vi "PNGout.vi"(2 "PNG file path":path=path "/Users/leogallacio/Downloads/N8.png", 7 "Paths error":errorcluster) -> (13 "PNGRead error":errorcluster, 14 "PNG picture":picture, 15 "Width":i16, 16 "Height":i16)   [LabVIEW 2023]
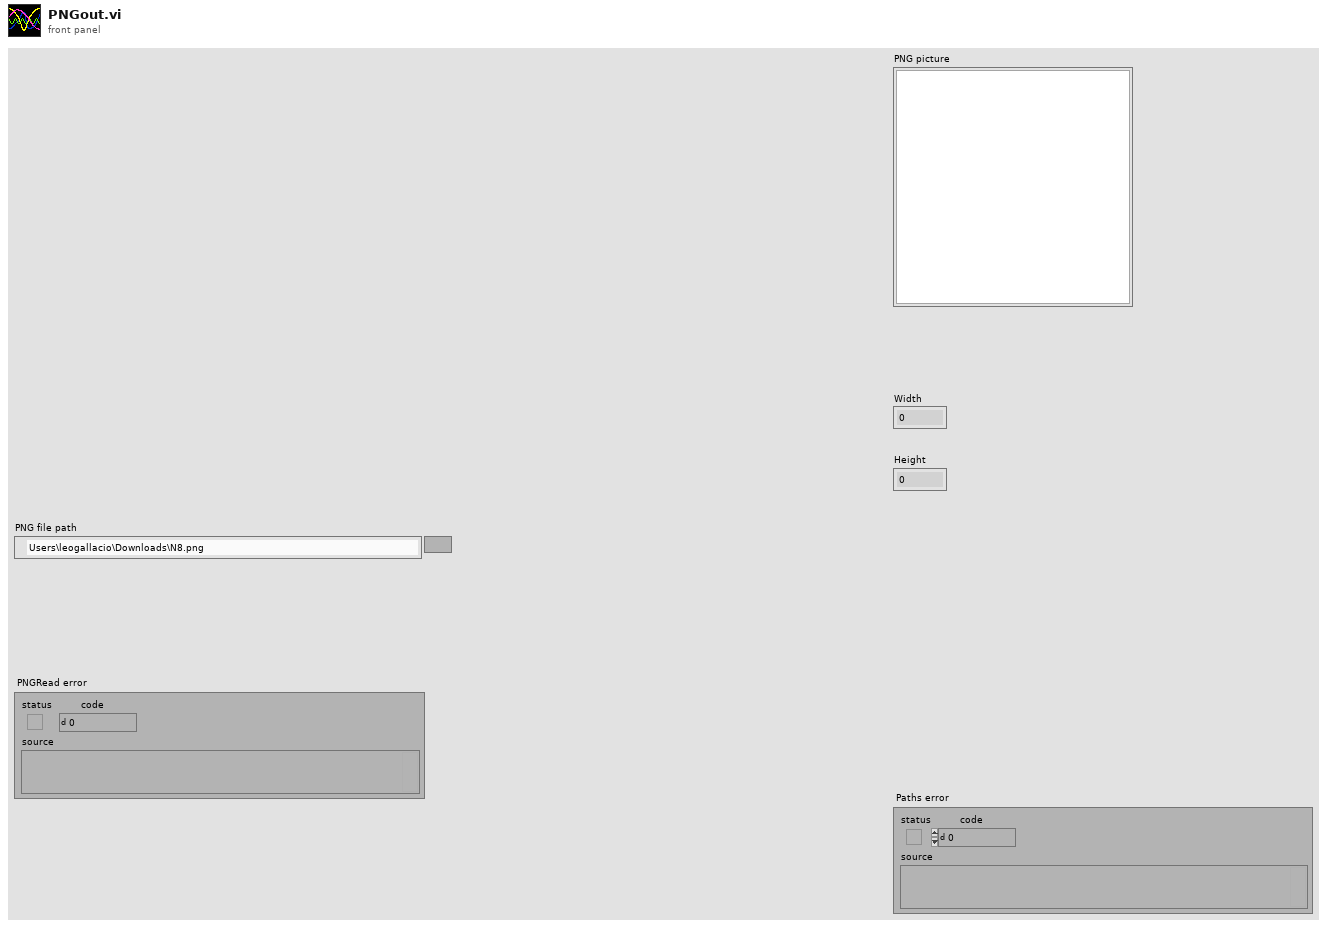
[diagram p1: front panel]
types:
  T1 = typedef "imagedata.ctl" = cluster{"image type":i32, "image depth":i32, "image":u8[], "mask":u8[], "colors":u32[], "Rectangle":cluster{"left":i16, "top":i16, "right":i16, "bottom":i16}}
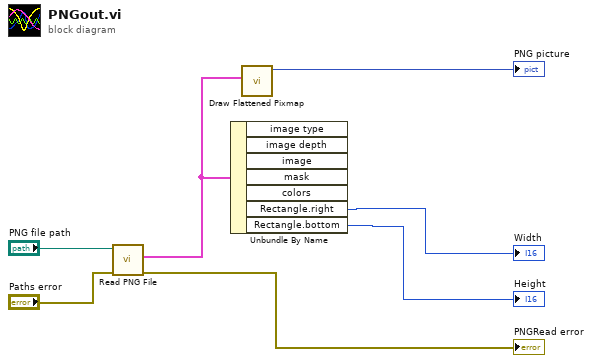
[diagram p0: block diagram]
diagram:
  n1 = call <vilib>:"Read PNG File.vi"("error in (no error)"="Paths error", "path to PNG file"="PNG file path") -> ("error out"=→"PNGRead error":errorcluster, "image data"=w5:T1)  [unwired: 7 in, 1 out]
  n2 = Unbundle By Name(w5) -> ("Rectangle.right"=→"Width":i16, "Rectangle.bottom"=→"Height":i16)  [unwired: 5 out]
  n3 = call <vilib>:"Draw Flattened Pixmap.vi"("image data"=w5) -> ("new picture"=→"PNG picture":picture)  [unwired: 8 in]
